vi "from string.vi"(8 "error in":errorcluster, 9 "data":string, 10 "version":string, 11 "CEF_Configuration in":refnum<class "CEF_serializable configuration.lvclass">) -> (0 "error out":errorcluster, 3 "CEF_Configuration out":refnum<class "CEF_serializable configuration.lvclass">)   [LabVIEW 2023, in "CEF.lvlib" / "CEF_serializable configuration.lvclass"]
doc: "Provides an interface for loading a module configuration from a file or other serialized data source. It is recommended that all children of this class store data in two sets--data required for its own initialization, and any data required for parent initialization--and that each implementation uses the <b>Call Parent Method</b> primitive to de-serialize parent information.Copyright 2017 National Instruments Corporation\n\nLicensed under the Apache License, Version 2.0 (the \"License\"); you may not use this file except in compliance with the License. You may obtain a copy of the License at http://www.apache.org/licenses/LICENSE-2.0\nUnless required by applicable law or agreed to in writing, software distributed under the License is distributed on an \"AS IS\" BASIS, WITHOUT WARRANTIES OR CONDITIONS OF ANY KIND, either express or implied. See the License for the specific language governing permissions and limitations under the License."
uses:
  CEF_serializable configuration.lvclass
  CEF_serializable configuration.lvclass/CEF_serializable configuration.ctl
  CEF.lvlib
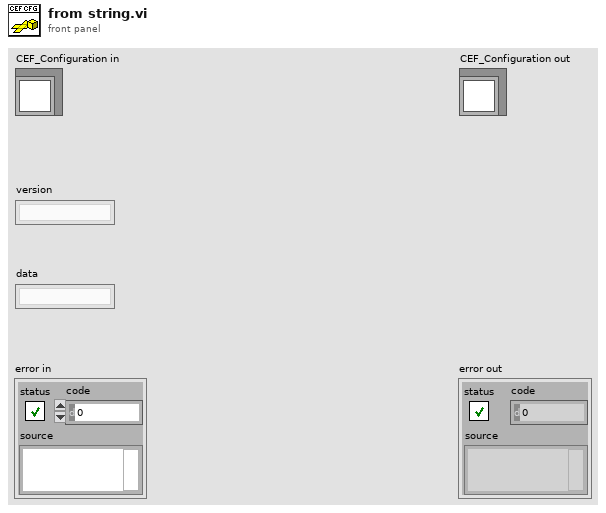
[diagram p1: front panel]
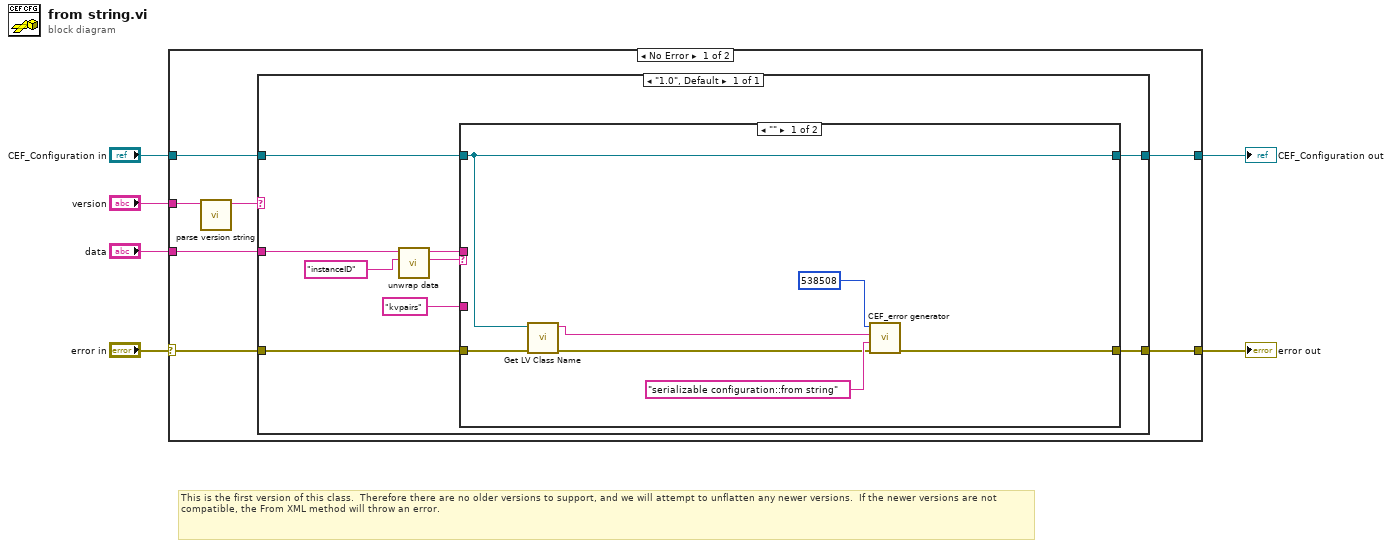
[diagram p0: block diagram]
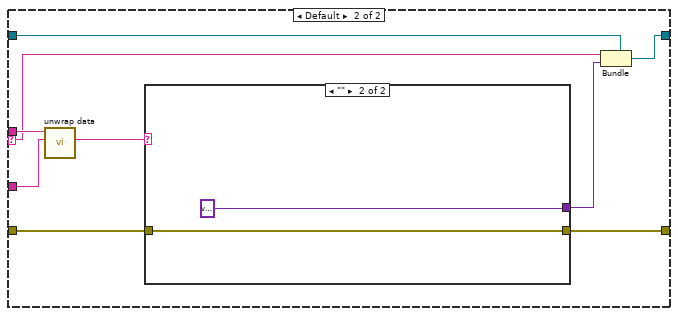
[diagram p2: hidden frame]
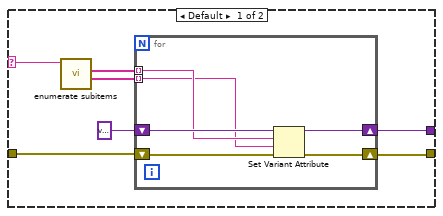
[diagram p3: hidden frame]
diagram:
  # "This is the first version of this class.  Therefore there are no older versions to support, and we will attempt to unflatten any newer versions.  If the newer versions are not compatible, the From XML method will throw an error."
  n1 = case shown="No Error" "error in" {
    selector: "error in" -> [w8 w55]
    tunnel: "data" -> [w13 _]
    tunnel: "CEF_Configuration in" -> [w12 w54]
    tunnel: [w11 w54] -> w1
    tunnel: [w7 w55] -> w2
    tunnel: "version" -> [w10 _]
    frame No Error {
      n2 = call "parse version string.vi"("full version"=w10) -> ("major.minor version"=w9:string)  [unwired: 7 in, 3 out]
      n3 = case shown="\"1.0\", Default" w9 {
        tunnel: w13 -> [w20]
        tunnel: w8 -> [w16]
        tunnel: w12 -> [w22]
        tunnel: [w21] -> w11
        tunnel: [w15] -> w7
        frame "1.0", Default {
          n4 = call "unwrap data.vi"("identifier"="instanceID" ("additional identifier"), "data to unwrap"=w20) -> ("unwrapped data"=w14:string, "remaining string"=w18:string)  [unwired: 8 in]
          n5 = case shown="\"\"" w14 {
            selector: w14 -> [_ w30]
            tunnel: w22 -> [w23 w38]
            tunnel: [w23 w37] -> w21
            tunnel: w18 -> [_ w36]
            tunnel: "kvpairs" ("additional identifier") -> [_ w35]
            tunnel: w16 -> [w26 w34]
            tunnel: [w29 w31] -> w15
            frame "" {
              n6 = call <vilib>:"Get LV Class Name.vi"("error in (no error)"=w26, "object"=w23) -> ("error out"=w25:errorcluster, "class name"=w24:string)  [unwired: 8 in]
              n7 = call "CEF_error generator.vi"("error in"=w25, "source"="serializable configuration::from string", "append error message"=w24, "error code (0)"=538508) -> ("error out"=w29:errorcluster)  [unwired: 5 in]
            }
            frame Default {
              n8 = call "unwrap data.vi"("identifier"=w35, "data to unwrap"=w36) -> ("unwrapped data"=w33:string)  [unwired: 8 in, 1 out]
              n9 = case shown="\"\"" w33 {
                selector: w33 -> [w42 _]
                tunnel: w34 -> [w41 w52]
                tunnel: [w44 variant ("key-value pairs")] -> w32
                tunnel: [w43 w52] -> w31
                frame Default {
                  n10 = call "enumerate subitems.vi"("data to enumerate"=w42) -> ("associated data"=w39:string[], "discovered subitems"=w40:string[])  [unwired: 8 in, 1 out]
                  n11 = for {
                    shift-right: [w50] -> w44
                    shift-left: variant ("key-value pairs") -> [w51]
                    shift-right: [w48] -> w43
                    shift-left: w41 -> [w49]
                    tunnel: w40 -> [w47] mode=indexing
                    tunnel: w39 -> [w46] mode=indexing
                    n12 = Set Variant Attribute(Variant=w51, name=w47, value=w46, error in=w49) -> (Variant out=w50:variant, error out=w48:errorcluster)  [unwired: 1 out]
                  }
                }
                frame "" {
                }
              }
              n13 = Bundle(cluster=w38, w30, w32) -> (w37:refnum<class "CEF_serializable configuration.lvclass">)
            }
          }
        }
      }
    }
    frame Error {
    }
  }
  "error out" <- w2
  "CEF_Configuration out" <- w1
